vi "set_gate_parameters.vi"(4 "repetition period":dbl[unit], 5 "offset":dbl[unit], 6 "number of repetitions":i64, 7 "clock index":i32, 8 "error in (no error)":errorcluster, 9 "pulsing frequency":dbl[unit], 10 "number of pulses":i64, 11 "GenericFPGAWrapper in":refnum<class "GenericFPGAWrapper.lvclass">) -> (0 "error out":errorcluster, 3 "GenericFPGAWrapper out":refnum<class "GenericFPGAWrapper.lvclass">)   [LabVIEW 2010, in "GenericFPGAWrapper.lvclass"]
doc: "Sets the timing parameters for the FPGA.\nclock index: which clock to set\noffset duration: delay until start of first train after \"start\" is issued\nhigh phase duration: duration, in which the gate is high (train of pulses)\nlow phase duration: output of pulses is supressed (pause)\npulse duration: period of the pulses (50% duty cycle)\nrepetitions: number of trains to issue"
uses:
  GenericFPGAWrapper.lvclass
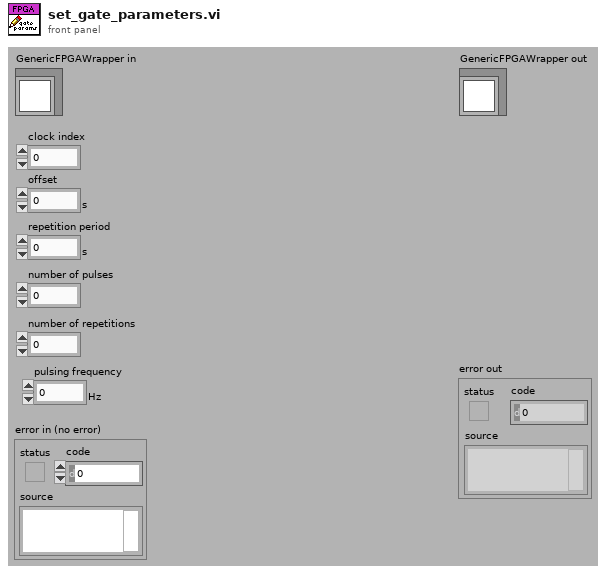
[diagram p1: front panel]
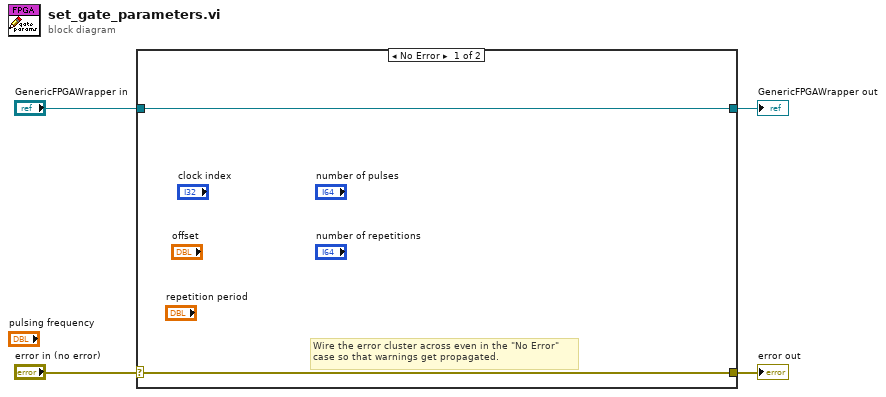
[diagram p0: block diagram]
diagram:
  n1 = case shown="No Error" "error in (no error)" {
    selector: "error in (no error)" -> [w5 w8]
    tunnel: [w5 w8] -> w3
    tunnel: [w6 w7] -> w1
    tunnel: "GenericFPGAWrapper in" -> [w6 w7]
    frame No Error {
      # "Wire the error cluster across even in the \"No Error\"\ncase so that warnings get propagated."
    }
    frame Error {
    }
  }
  "error out" <- w3
  "GenericFPGAWrapper out" <- w1
